vi "Blocker logic.vi"(11 "Botton on":bool) -> ()   [LabVIEW 2013]
uses:
  <vilib>/Rock Robotics/WPI/Relay/WPI_RelayValue.ctl
panel:
  in  "Blocker State":enum16{"Going Up", "Up", "Going Down", "Down"}(ring)
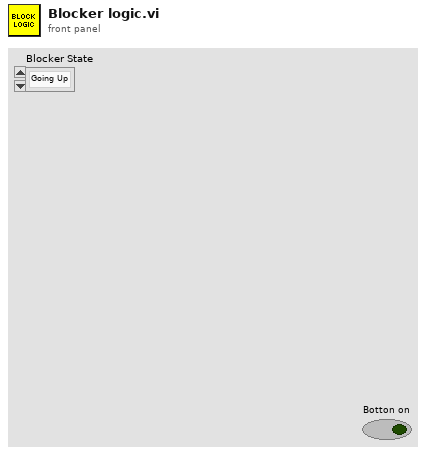
[diagram p1: front panel]
types:
  T1 = typedef "WPI_RelayValue.ctl" = enum16{"Off", "On", "Forward", "Reverse"}
  T2 = typedef "WPI_DigitalInputDevRef.ctl" = cluster{"DevStatus":errorcluster, "DIO Channel":T3, "Digital Module":T4}
  T3 = typedef "FPGA_DIOChannel.ctl" = enum8{"DIO 1", "DIO 2", "DIO 3", "DIO 4", "DIO 5", "DIO 6", "DIO 7", "DIO 8", "DIO 9", "DIO 10", "DIO 11", "DIO 12", "DIO 13", "DIO 14", "Invalid"}
  T4 = typedef "FPGA_TypedefDigitalModule.ctl" = enum16{"Digital Module 1", "Digital Module 2"}
  T5 = typedef "WPI_RelayDevRef.ctl" = cluster{"DevStatus":errorcluster, "Relay Channel":T6, "Digital Module":T4, "Relay Direction":T7}
  T6 = typedef "FPGA_DIORelayChannel.ctl" = enum8{"Relay 1", "Relay 2", "Relay 3", "Relay 4", "Relay 5", "Relay 6", "Relay 7", "Relay 8", "Invalid"}
  T7 = typedef "WPI_RelayDirection.ctl" = enum16{"Both directions", "Forward only", "Reverse only"}
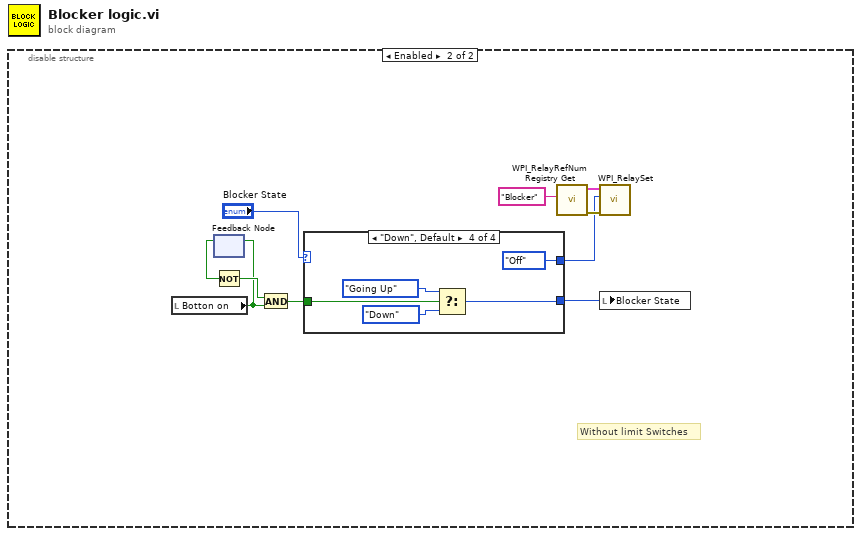
[diagram p0: block diagram]
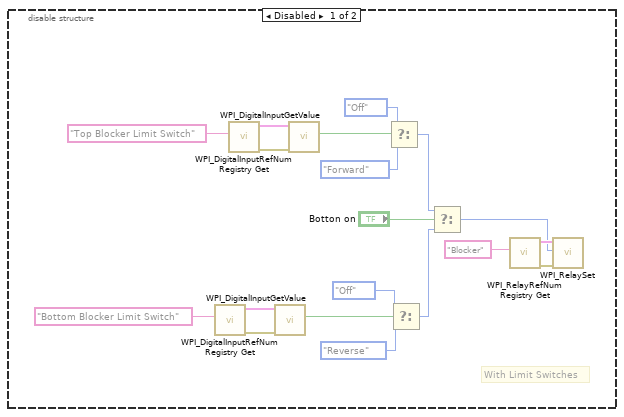
[diagram p2: hidden frame]
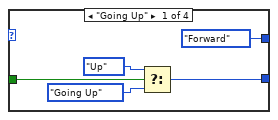
[diagram p3: hidden frame]
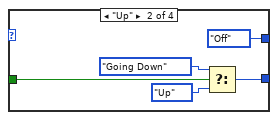
[diagram p4: hidden frame]
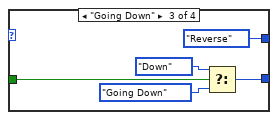
[diagram p5: hidden frame]
diagram:
  n1 = disable-structure shown="Enabled" {
    frame Disabled {
      # "With Limit Switches"
      n2 = call <vilib>:"WPI_DigitalInputRefNum Registry Get.vi"("refnum name"="Bottom Blocker Limit Switch") -> ("error out"=w4:errorcluster, "DigitalInputDevRef"=w3:T2)  [unwired: 9 in]
      n3 = call <vilib>:"WPI_DigitalInputRefNum Registry Get.vi"("refnum name"="Top Blocker Limit Switch") -> ("error out"=w8:errorcluster, "DigitalInputDevRef"=w7:T2)  [unwired: 9 in]
      n4 = call <vilib>:"WPI_DigitalInputGetValue.vi"("error in (no error)"=w4, "DigitalInputDevRef"=w3) -> ("Value"=w1:bool)  [unwired: 7 in, 2 out]
      n5 = call <vilib>:"WPI_DigitalInputGetValue.vi"("error in (no error)"=w8, "DigitalInputDevRef"=w7) -> ("Value"=w5:bool)  [unwired: 7 in, 2 out]
      n6 = Select(t=WPI_RelayValue."Off" ("Blocker State"), s=w5, f=WPI_RelayValue."Forward" ("Blocker State")) -> (s? t:f=w13:T1)
      n7 = Select(t=WPI_RelayValue."Off" ("Blocker State"), s=w1, f=WPI_RelayValue."Reverse" ("Blocker State")) -> (s? t:f=w10:T1)
      n8 = Select(t=w13, s="Botton on", f=w10) -> (s? t:f=w9:T1)
      n9 = call <vilib>:"WPI_RelayRefNum Registry Get.vi"("refnum name"="Blocker") -> ("error out"=w19:errorcluster, "RelayDevRef"=w18:T5)  [unwired: 9 in]
      n10 = call <vilib>:"WPI_RelaySet.vi"("error in (no error)"=w19, "RelayValue"=w9, "RelayDevRef"=w18) -> ()  [unwired: 7 in, 2 out]
    }
    frame Enabled {
      # "Without limit Switches"
      n11 = local read "Botton on"() -> (w22:bool)
      n12 = feedback-in #1(w22) -> ()
      n13 = feedback #1() -> (w24:bool)  [unwired: 1 in]
      n14 = Not(x=w24) -> (.not. x?=w23:bool)
      n15 = And(x=w23, y=w22) -> (x .and. y?=w21:bool)
      n16 = case shown="\"Down\", Default" "Blocker State" {
        tunnel: [WPI_RelayValue."Forward" ("RelayValue") WPI_RelayValue."Off" ("RelayValue") WPI_RelayValue."Reverse" ("RelayValue") WPI_RelayValue."Off" ("RelayValue")] -> w25
        tunnel: w21 -> [w31 w36 w41 w48]
        tunnel: [w30 w35 w40 w45] -> w20
        frame "Going Up" {
          n17 = Select(t=enum16{"Going Up", "Up", "Going Down", "Down"}."Up", s=w31, f=enum16{"Going Up", "Up", "Going Down", "Down"}."Going Up") -> (s? t:f=w30:enum16{"Going Up", "Up", "Going Down", "Down"})
        }
        frame "Up" {
          n18 = Select(t=enum16{"Going Up", "Up", "Going Down", "Down"}."Going Down", s=w36, f=enum16{"Going Up", "Up", "Going Down", "Down"}."Up") -> (s? t:f=w35:enum16{"Going Up", "Up", "Going Down", "Down"})
        }
        frame "Going Down" {
          n19 = Select(t=enum16{"Going Up", "Up", "Going Down", "Down"}."Down", s=w41, f=enum16{"Going Up", "Up", "Going Down", "Down"}."Going Down") -> (s? t:f=w40:enum16{"Going Up", "Up", "Going Down", "Down"})
        }
        frame "Down", Default {
          n20 = Select(t=enum16{"Going Up", "Up", "Going Down", "Down"}."Going Up", s=w48, f=enum16{"Going Up", "Up", "Going Down", "Down"}."Down") -> (s? t:f=w45:enum16{"Going Up", "Up", "Going Down", "Down"})
        }
      }
      n21 = call <vilib>:"WPI_RelayRefNum Registry Get.vi"("refnum name"="Blocker") -> ("error out"=w26:errorcluster, "RelayDevRef"=w27:T5)  [unwired: 9 in]
      n22 = call <vilib>:"WPI_RelaySet.vi"("error in (no error)"=w26, "RelayValue"=w25, "RelayDevRef"=w27) -> ()  [unwired: 7 in, 2 out]
      n23 = local write "Blocker State"(w20) -> ()
    }
  }
